vi "Create Execution Unit.vi"(8 "error in":errorcluster, 10 "Custom Device Ref":T2=18446744073709551615 format="%.0x", 11 "Execution Unit Factory Implementation in":refnum<class "Execution Unit Factory.lvclass">) -> (0 "error out":errorcluster, 1 "Asynchronous Execution Units":T1[](array[typedef]) {"ReadWrite Channels" format="%.0x"; "Outgoing Channels" format="%.0x"; "Incoming Channels" format="%.0x"}, 2 "Inline Execution Units":T1[](array[typedef]) {"ReadWrite Channels" format="%.0x"; "Outgoing Channels" format="%.0x"; "Incoming Channels" format="%.0x"}, 3 "Execution Unit Factory Implementation out":refnum<class "Execution Unit Factory.lvclass">)   [LabVIEW 2020, in "AIM ARINC 664 Engine.lvlib" / "Implementation.lvlib" / "Execution Unit Factory.lvclass"]
uses:
  Execution Unit Factory.lvclass
  <vilib>/NI VeriStand/Custom Device API/Custom Device Item Ref.ctl
  Interfaces/Controls/Execution Unit Information.ctl
  Interfaces/Execution Unit/Execution Unit.lvclass
  Tx Execution Unit/Tx Generic Execution Unit.lvclass
  C:/Users/Administrator/Desktop/GIT/niveristand-aim-arinc664-custom-device/Source/Custom Device Support/Engine/Interfaces/Execution Unit/Execution Unit.lvclass
  Tx UDP Execution Unit/Tx UDP Execution Unit.lvclass
  Rx UDP Execution Unit/Rx UDP Execution Unit.lvclass
  Monitor Execution Unit/Monitor Execution Unit.lvclass
  <vilib>/NI VeriStand/Custom Device API/Custom Device API.lvlib
  Interfaces/Interfaces.lvlib
  Scripting/AIM ARINC 664 Scripting.lvlib
  <vilib>/Utility/SystemLogging/NI_SystemLogging.lvlib
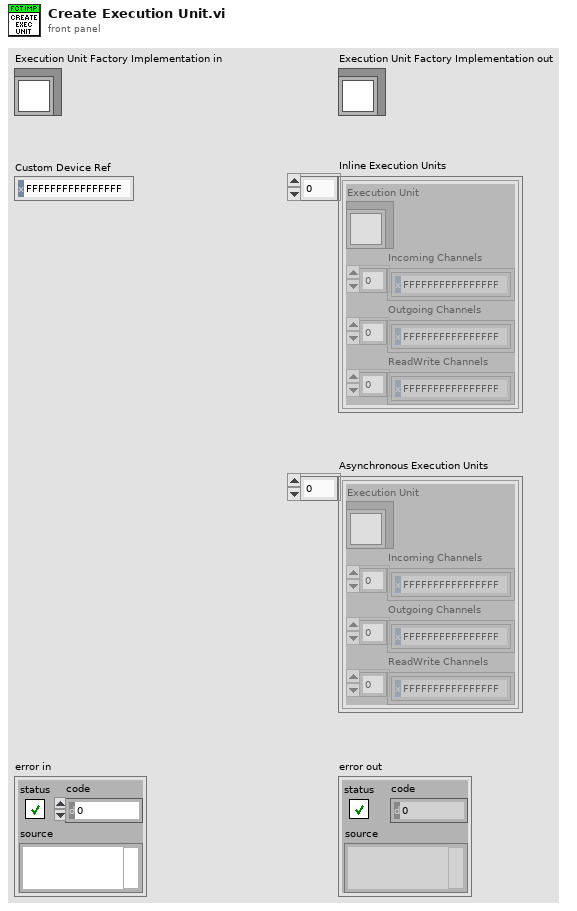
[diagram p1: front panel]
types:
  T1 = typedef "AIM ARINC 664 Engine.lvlib/Interfaces.lvlib/Execution Unit Information.ctl" = cluster{"Execution Unit":refnum<class "Execution Unit.lvclass">, "Incoming Channels":T2[], "Outgoing Channels":T2[], "ReadWrite Channels":T2[]}
  T2 = typedef "Custom Device API.lvlib/Custom Device Item Ref.ctl" = u64
  T3 = typedef "Custom Device API.lvlib/Custom Device Target Type.ctl" = enum16{"PharLap", "VxWorks", "Windows", "Linux_32_ARM", "Linux_x64"}
  T4 = typedef "AIM ARINC 664 Import.lvlib/board_setup.ctl" = cluster{"boardId":u32, "portSpeed":u32, "portConfig":u32}
  T5 = typedef "AIM ARINC 664 Import.lvlib/port_setup.ctl" = cluster{"port Id":u32, "redundant":bool}
  T6 = typedef "hardware_channels_tx.ctl" = cluster{"channel #":u16, "channel handle":u64, "InstrumentHandle_board":u32, "InstrumentHandle_port":u32, "channel settings":T7, "PayloadMap":map{string, u8[]}, "RawFrameMap":map{string, T10}}
  T7 = typedef "channel_settings_tx.ctl" = cluster{"Tx Board":u32, "Tx Port":u32, "Payload Parameter Array":T8[], "QueueSizeIn":u32, "Count":u32, "StartMode":u32}
  T8 = typedef "Frame Payload Parameters.ctl" = cluster{"PayloadID":string, "FrameIndeces":u32[], "Parameters":cluster{"start index":i32, "size":i32, "encoding":T9, "signed":bool, "scale multiplier":dbl, "scale offset":dbl}[]}
  T9 = typedef "Encoding (Arinc664).ctl" = u16
  T10 = typedef "RawFrame_entry.ctl" = cluster{"HeaderInfo":T11, "PayloadID":string}
  T11 = typedef "AIM664LV.lvlib/queue_header_generic.ctl" = cluster{"InterFrameGap":u32, "PacketGroupWaitTime":u32, "PayloadBufferMode":u8, "PayloadGenerationMode":u8, "PreambleCount":u8, "Skew":u32, "NetSelect":u8, "FrameStartMode":u8, "PhysErrorInjection":u32, "SequenceNumberInit":u16, "SequenceNumberOffset":u16}
  T12 = typedef "AIM664LV.lvlib/comm_config_vl_tx.ctl" = cluster{"VlId":u16, "NumOfSubVl":u16, "rate ms [Bag]":u32, "domainID":u8, "sideID":u8, "locationID":u8, "interfaceID":u8, "NetSelect":u32, "Skew":u32, "MaxFrameLength":u32, "FrameBufferSize":u32}
  T13 = typedef "AIM664LV.lvlib/comm_udp_tx.ctl" = cluster{"PortType":enum16{"FDX_UDP_SAMPLING", "FDX_UDP_QUEUING"}, "partitionID":u8, "SubVlId":u8, "UdpSrcPort":u16, "UdpDstPort":u16, "SampleRateMs":dbl, "UdpNumBufMessages":u32, "UdpMaxMessageSize":u32}
  T14 = cluster{"VL Config":T12, "CommPort Config":T13[]}[]
  T15 = cluster{"Data":u8[], "Parameters":cluster{"start index":i32, "size":i32, "encoding":T9, "signed":bool, "scale multiplier":dbl, "scale offset":dbl}[]}[]
  T16 = typedef "AIM664LV.lvlib/comm_verification_rx.ctl" = cluster{"VlId":u16, "VLRange":u32, "VerificationMode":u32, "Bag":u32, "Jitter":u32, "MaxFrameLength":u32, "MaxSkew":u32, "VLBufSize":u32, "FilterMode":u32, "FilterPosition":u32, "Padding":u32, "FilterMask":u32, "FilterData":u32, "MinFrameLength":u32}
  T17 = typedef "AIM664LV.lvlib/comm_udp_rx.ctl" = cluster{"PortType":enum16{"FDX_UDP_SAMPLING", "FDX_UDP_QUEUING"}, "SubVIId":u32, "domainID":u8, "sideID":u8, "locationID":u8, "partitionID":u8, "UdpSrcPort":u16, "UdpDstPort":u16, "UdpNumBufMessages":u32, "UdpMaxMessageSize":u32, "UdpSamplingRate":u32}
  T18 = cluster{"VL Config":T16, "CommPort Config":T17[]}[]
  T19 = typedef "rx_udp_payload_config.ctl" = cluster{"Data":u8[], "Parameters":cluster{"start index":i32, "size":i32, "encoding":T9, "signed":bool, "scale multiplier":dbl, "scale offset":dbl}[], "GetStatus":bool}
  T20 = typedef "loggingThreshold_types.ctl" = cluster{"Segmentation Threshold":dbl, "Disk Space Percentage":dbl, "Check Disk Space":bool, "Segment File":bool, "Segment Files By":u16}
  T21 = typedef "logFileInfo_types.ctl" = cluster{"Log Directory":string, "Base Name":string, "Timestamp":bool, "Enabled":bool}
  T22 = typedef "hardware_channels_rx.ctl" = cluster{"channel #":u16, "channel handle":u64, "InstrumentHandle_board":u32, "InstrumentHandle_port":u32, "Queue ID":u32, "channel settings":T23, "current log file name":path, "monitor queue settings":T25, "Log File Directory":string, "Base name":string, "Timestamp":bool, "log thresholds":T20}
  T23 = typedef "channel_settings_rx.ctl" = cluster{"Monitor Settings":T24, "Rx Board":u32, "Rx Port":u32}
  T24 = typedef "AIM664LV.lvlib/session_monitor_config.ctl" = cluster{"DefaultCronoMode":u32, "GlbMonBufferSizeIn":u32}
  T25 = typedef "monitor_queue_settings.ctl" = cluster{"TriggerPosition":u32, "CaptureMode":u32, "Strobe":u32, "MaxFileSize MB (1)":u32}
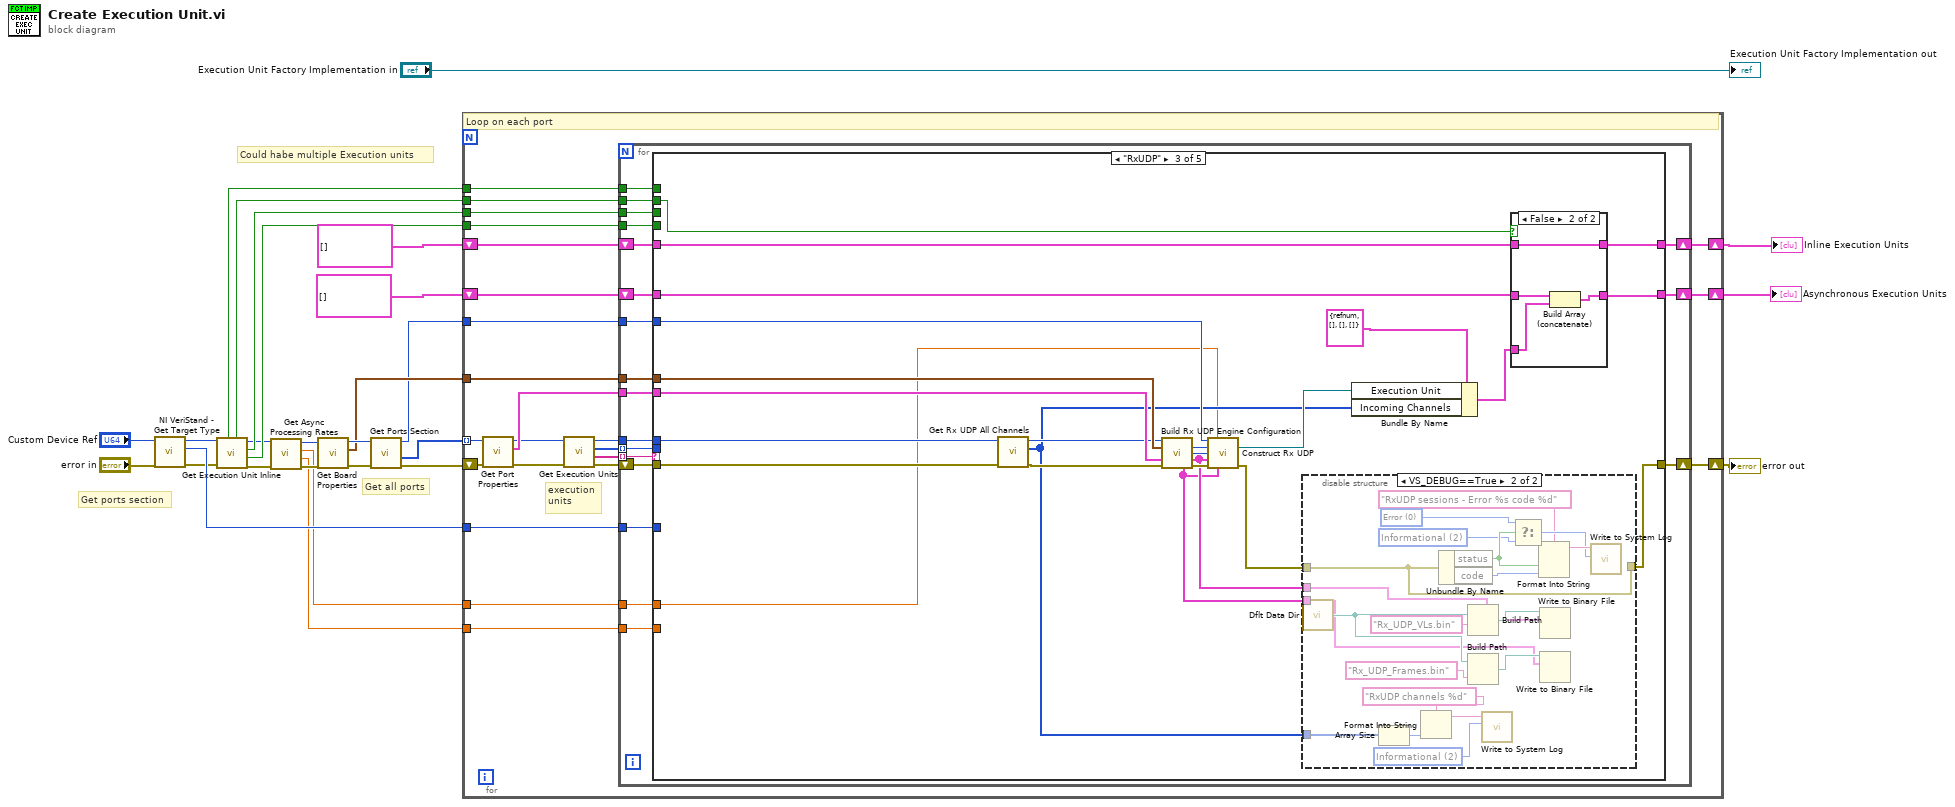
[diagram p0: block diagram]
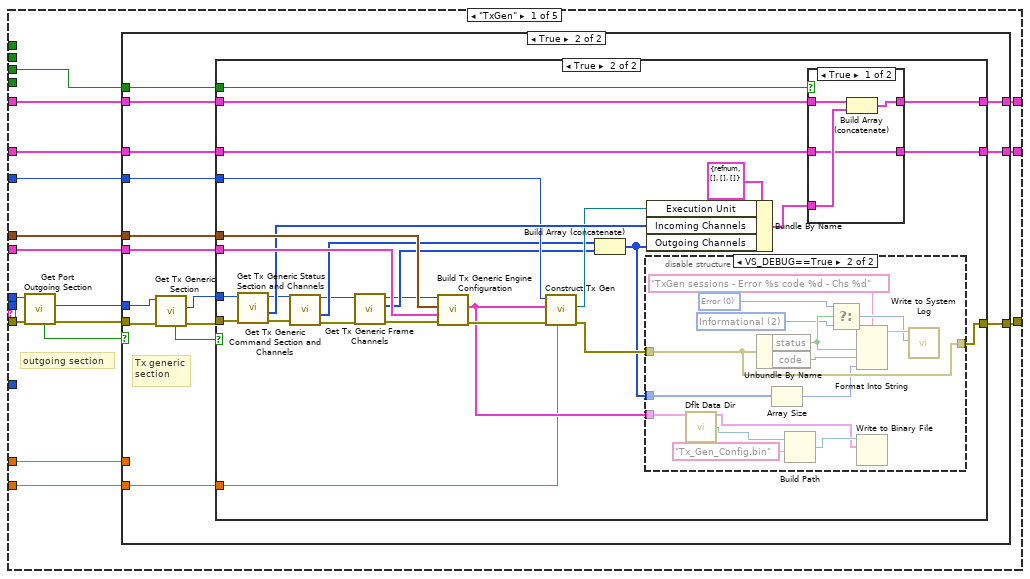
[diagram p2: hidden frame]
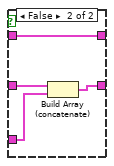
[diagram p5: hidden frame]
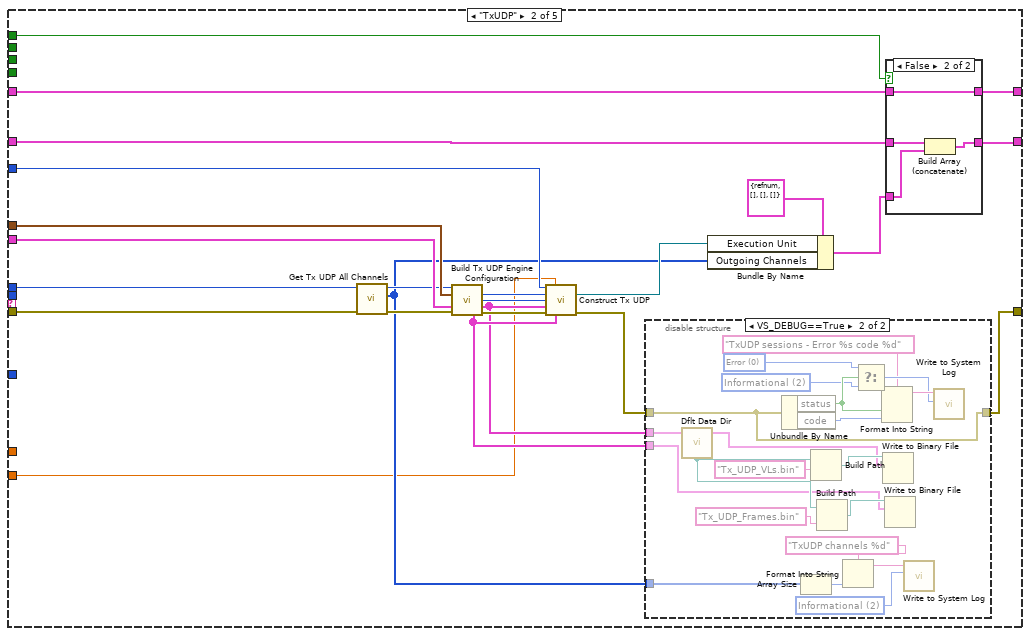
[diagram p7: hidden frame]
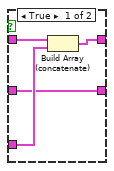
[diagram p8: hidden frame]
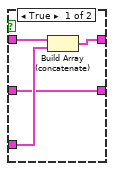
[diagram p10: hidden frame]
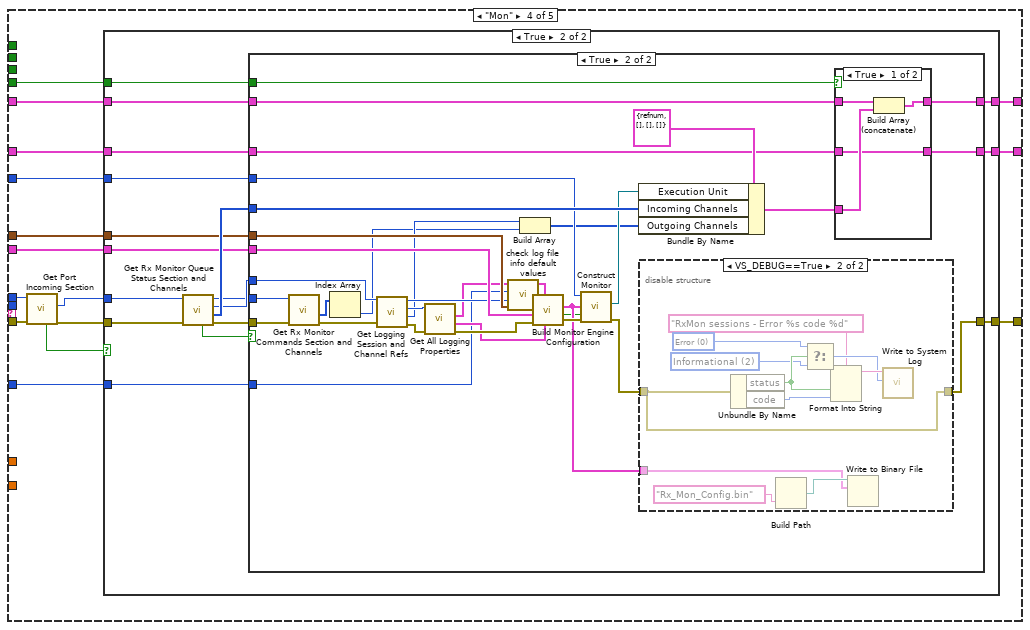
[diagram p12: hidden frame]
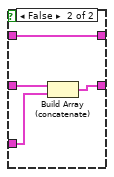
[diagram p15: hidden frame]
diagram:
  # "Get all ports"
  # "Get ports section"
  # "Could habe multiple Execution units"
  n1 = call <vilib>:"NI VeriStand - Get Target Type.vi"("error in (no error)"="error in", "Item Ref in"="Custom Device Ref") -> ("error out"=w12:errorcluster, "Target Type"=w13:T3, "Item Ref out"=w11:T2)  [unwired: 7 in]
  n2 = call "Get Execution Unit Inline.vi"("error in"=w12, "custom device ref"=w11) -> ("error out"=w5:errorcluster, "Inline Rx Execution"=w8:bool, "Inline Tx Generic"=w10:bool, "custom device ref out"=w6:T2, "Inline Rx UDP"=w7:bool, "Inline Tx UDP"=w9:bool)  [unwired: 4 in]
  n3 = call "Get Async Processing Rates.vi"("error in"=w5, "custom device ref"=w6) -> ("error out"=w4:errorcluster, "Outgoing Frame Rate"=w2:dbl, "Incoming Frame Rate"=w1:dbl, "custom device ref out"=w3:T2)  [unwired: 6 in]
  n4 = call "Get Board Properties.vi"("error in"=w4, "custom device ref"=w3) -> ("error out"=w21:errorcluster, "board properties out"=w19:T4, "custom device ref out"=w20:T2)  [unwired: 7 in]
  n5 = call "Get Ports Section.vi"("error in"=w21, "custom device ref"=w20) -> ("error out"=w18:errorcluster, "all ports refs out"=w17:T2[], "custom device ref out"=w16:T2)  [unwired: 6 in, 1 out]
  n6 = for {
    shift-right: [w46] -> w26
    shift-left: w18 -> [w43]
    tunnel: w17 -> [w44] mode=indexing
    shift-right: [w48] -> w22
    shift-left: T1[] [] ("Array") -> [w49]
    shift-right: [w47] -> w23
    shift-left: T1[] [] ("Array") -> [w50]
    tunnel: w19 -> [w45]
    tunnel: w16 -> [w41]
    tunnel: w13 -> [w34]
    tunnel: w10 -> [w33]
    tunnel: w9 -> [w32]
    tunnel: w8 -> [w31]
    tunnel: w7 -> [w30]
    tunnel: w2 -> [w29]
    tunnel: w1 -> [w28]
    # "execution\nunits"
    # "Loop on each port"
    n7 = call "Get Port Properties.vi"("error in"=w43, "custom device ref"=w44) -> ("error out"=w39:errorcluster, "port properties out"=w42:T5, "custom device ref out"=w40:T2)  [unwired: 7 in]
    n8 = call "Get Execution Units.vi"("error in"=w39, "custom device ref"=w40) -> ("error out"=w37:errorcluster, "List of Execution Units"=w35:string[], "Execution Units Refs"=w36:T2[], "custom device ref out"=w38:T2)  [unwired: 6 in]
    n9 = for {
      tunnel: w38 -> [w68]
      shift-right: [w63] -> w46
      shift-left: w37 -> [w69]
      shift-right: [w64] -> w47
      shift-left: w50 -> [w67]
      shift-right: [w65] -> w48
      shift-left: w49 -> [w66]
      tunnel: w42 -> [w62]
      tunnel: w45 -> [w61]
      tunnel: w41 -> [w60]
      tunnel: w36 -> [w58] mode=indexing
      tunnel: w35 -> [w59] mode=indexing
      tunnel: w34 -> [w57]
      tunnel: w33 -> [w56]
      tunnel: w32 -> [w55]
      tunnel: w31 -> [w54]
      tunnel: w30 -> [w53]
      tunnel: w29 -> [w52]
      tunnel: w28 -> [w51]
      n10 = case shown="\"RxUDP\"" w59 {
        tunnel: w69 -> [w85 w181 w234 w278 w355]
        tunnel: w68 -> [w84 w170 w223 w277 _]
        tunnel: w67 -> [w80 w162 w216 w273 w357]
        tunnel: w66 -> [w79 w164 w214 w272 w356]
        tunnel: [w77 w159 w213 w271 w356] -> w65
        tunnel: [w78 w160 w217 w270 w357] -> w64
        tunnel: [w76 w166 w219 w269 w355] -> w63
        tunnel: w62 -> [w75 w175 w228 w267 _]
        tunnel: w61 -> [w74 w176 w229 w268 _]
        tunnel: w60 -> [w73 w171 w224 w266 _]
        tunnel: w58 -> [_ _ _ _ _]
        tunnel: w57 -> [_ _ _ w265 _]
        tunnel: w56 -> [w72 _ _ _ _]
        tunnel: w55 -> [_ w161 _ _ _]
        tunnel: w54 -> [_ _ _ w264 _]
        tunnel: w53 -> [_ _ w212 _ _]
        tunnel: w52 -> [w71 w158 _ _ _]
        tunnel: w51 -> [w70 _ w211 _ _]
        frame "TxGen" {
          # "outgoing section"
          n11 = call "Get Port Outgoing Section.vi"("error in"=w85, "ports ref"=w84) -> ("error out"=w82:errorcluster, "outgoing section ref out"=w81:T2, "found?"=w83:bool)  [unwired: 6 in, 1 out]
          n12 = case shown="True" w83 {
            tunnel: w82 -> [w86 w96]
            tunnel: w81 -> [_ w95]
            tunnel: w80 -> [w88 w102]
            tunnel: w79 -> [w87 w101]
            tunnel: [w88 w103] -> w78
            tunnel: [w87 w100] -> w77
            tunnel: [w86 w99] -> w76
            tunnel: w75 -> [_ w98]
            tunnel: w74 -> [_ w97]
            tunnel: w73 -> [_ w91]
            tunnel: w72 -> [_ w90]
            tunnel: w71 -> [_ w89]
            tunnel: w70 -> [_ _]
            frame False {
            }
            frame True {
              # "Tx generic\nsection"
              n13 = call "Get Tx Generic Section.vi"("error in"=w96, "Parent section Ref in"=w95) -> ("error out"=w93:errorcluster, "Item Ref"=w92:T2, "found?"=w94:bool)  [unwired: 6 in, 1 out]
              n14 = case shown="True" w94 {
                tunnel: w93 -> [w104 w128]
                tunnel: [w106 w112] -> w103
                tunnel: w102 -> [w106 w133]
                tunnel: w101 -> [w105 w132]
                tunnel: [w105 w110] -> w100
                tunnel: [w104 w118] -> w99
                tunnel: w98 -> [_ w130]
                tunnel: w97 -> [_ w129]
                tunnel: w92 -> [_ w127]
                tunnel: w91 -> [_ w124]
                tunnel: w90 -> [_ w108]
                tunnel: w89 -> [_ w107]
                frame False {
                }
                frame True {
                  n15 = call "Get Tx Generic Status Section and Channels.vi"("error in"=w128, "Tx generic ref"=w127) -> ("error out"=w122:errorcluster, "Tx generic status channel refs"=w126:T2[], "Tx generic ref out"=w123:T2)  [unwired: 5 in, 2 out]
                  n16 = call "Get Tx Generic Command Section and Channels.vi"("error in"=w122, "Tx generic ref"=w123) -> ("error out"=w117:errorcluster, "Tx generic command channel refs"=w121:T2[], "Tx generic ref out"=w116:T2)  [unwired: 5 in, 2 out]
                  n17 = call "Get Tx Generic Frame Channels.vi"("error in"=w117, "Tx generic ref"=w116) -> ("error out"=w115:errorcluster, "Tx generic frame channels"=w114:T2[], "Tx generic ref out"=w113:T2)  [unwired: 6 in, 1 out]
                  n18 = call "Build Tx Generic Engine Configuration.vi"("error in"=w115, "port properties"=w130, "board properties"=w129, "section ref in"=w113) -> ("error out"=w131:errorcluster, "Tx cluster out"=w119:T6)  [unwired: 5 in, 1 out]
                  n19 = call "Construct Tx Gen.vi"("async loop rate hz"=w107, "error in (no error)"=w131, "TX Parameters"=w119, "custom device ref in"=w124) -> ("error out"=w120:errorcluster, "Tx Execution Unit out"=w125:refnum<class "Tx Generic Execution Unit.lvclass">)  [unwired: 4 in, 1 out]
                  n20 = Build Array (concatenate)(w121, w114) -> (w111:T2[])
                  n21 = disable-structure shown="VS_DEBUG==True" {
                    disable-tunnel: w120 -> [w143 w146]
                    disable-tunnel: w119 -> [_ w147]
                    disable-tunnel: [w143 w146] -> w118
                    disable-tunnel: w111 -> [_ w145]
                    frame condition #0 (active) {
                    }
                    frame condition #1 {
                      w153 = 2 items=["Error", "Warning", "Informational"] ("severity")
                      w154 = 0 items=["Error", "Warning", "Informational"] ("severity")
                      n22 = call <vilib>:"Dflt Data Dir.vi"() -> ("App:Default Data Directory"=w150:path)
                      n23 = Unbundle By Name(w146) -> ("status"=w155:bool, "code"=w156:i32)
                      n24 = Array Size(array=w145) -> (size(s)=w144:i32)
                      n25 = Build Path(base path=w150, name or relative path="Tx_Gen_Config.bin" ("format string")) -> (appended path=w148:path)
                      n26 = Select(t=w154, s=w155, f=w153) -> (s? t:f=w152:i32)
                      n27 = Format Into String(format string="TxGen sessions - Error %s code %d - Chs %d", w155, w156, w144) -> (resulting string=w157:string)  [unwired: 2 in, 1 out]
                      n28 = Write to Binary File(file (use dialog)=w148, data=w147) -> ()  [unwired: 4 in, 3 out]
                      n29 = call <vilib>:"Write to System Log.vi"("severity"=w152, "message"=w157) -> ()  [unwired: 9 in, 1 out]
                    }
                  }
                  n30 = Bundle By Name(cluster=T1 {"Execution Unit"=refnum, "Incoming Channels"=[], "Outgoing Channels"=[], "ReadWrite Channels"=[]} ("Execution Unit Information"), "Execution Unit"=w125, "Incoming Channels"=w126, "Outgoing Channels"=w111) -> (w109:T1)
                  n31 = case shown="True" w108 {
                    tunnel: w133 -> [w138 w142]
                    tunnel: w132 -> [w135 w141]
                    tunnel: [w137 w142] -> w112
                    tunnel: [w135 w140] -> w110
                    tunnel: w109 -> [w136 w139]
                    frame True {
                      n32 = Build Array (concatenate)(w138, w136) -> (w137:T1[])
                    }
                    frame False {
                      n33 = Build Array (concatenate)(w141, w139) -> (w140:T1[])
                    }
                  }
                }
              }
            }
          }
        }
        frame "TxUDP" {
          n34 = call "Get Tx UDP All Channels.vi"("error in"=w181, "custom device ref in"=w170) -> ("error out"=w178:errorcluster, "Tx UDP channel refs out"=w165:T2[], "custom device ref out"=w172:T2)  [unwired: 7 in]
          n35 = call "Build Tx UDP Engine Configuration.vi"("section ref in"=w172, "board properties"=w176, "port properties"=w175, "error in"=w178) -> ("boardId"=w174:u32, "portId"=w173:u32, "VL configurations"=w167:T14, "comm port payload"=w168:T15, "error out"=w177:errorcluster)  [unwired: 6 in, 1 out]
          n36 = call "Construct Tx UDP.vi"("custom device ref in"=w171, "async loop rate hz"=w158, "InstrumentHandle_board"=w174, "InstrumentHandle_port"=w173, "VL Configurations"=w167, "error in (no error)"=w177, "CommPort Payload"=w168) -> ("Execution Unit Out"=w179:refnum<class "Tx UDP Execution Unit.lvclass">, "error out"=w169:errorcluster)  [unwired: 6 in, 1 out]
          n37 = disable-structure shown="VS_DEBUG==True" {
            disable-tunnel: w169 -> [w190 w196]
            disable-tunnel: w168 -> [_ w197]
            disable-tunnel: w167 -> [_ w198]
            disable-tunnel: [w190 w196] -> w166
            disable-tunnel: w165 -> [_ w193]
            frame condition #0 (active) {
            }
            frame condition #1 {
              w191 = 2 items=["Error", "Warning", "Informational"] ("severity")
              w206 = 2 items=["Error", "Warning", "Informational"] ("severity")
              w207 = 0 items=["Error", "Warning", "Informational"] ("severity")
              n38 = call <vilib>:"Dflt Data Dir.vi"() -> ("App:Default Data Directory"=w203:path)
              n39 = Unbundle By Name(w196) -> ("status"=w208:bool, "code"=w209:i32)
              n40 = Array Size(array=w193) -> (size(s)=w195:i32)
              n41 = Build Path(base path=w203, name or relative path="Tx_UDP_VLs.bin" ("format string")) -> (appended path=w200:path)
              n42 = Build Path(base path=w203, name or relative path="Tx_UDP_Frames.bin" ("format string")) -> (appended path=w199:path)
              n43 = Format Into String(format string="TxUDP channels %d", w195) -> (resulting string=w194:string)  [unwired: 2 in, 1 out]
              n44 = Select(t=w207, s=w208, f=w206) -> (s? t:f=w205:i32)
              n45 = Format Into String(format string="TxUDP sessions - Error %s code %d", w208, w209) -> (resulting string=w210:string)  [unwired: 2 in, 1 out]
              n46 = Write to Binary File(file (use dialog)=w200, data=w198) -> ()  [unwired: 4 in, 3 out]
              n47 = Write to Binary File(file (use dialog)=w199, data=w197) -> ()  [unwired: 4 in, 3 out]
              n48 = call <vilib>:"Write to System Log.vi"("severity"=w191, "message"=w194) -> ()  [unwired: 9 in, 1 out]
              n49 = call <vilib>:"Write to System Log.vi"("severity"=w205, "message"=w210) -> ()  [unwired: 9 in, 1 out]
            }
          }
          n50 = Bundle By Name(cluster=T1 {"Execution Unit"=refnum, "Incoming Channels"=[], "Outgoing Channels"=[], "ReadWrite Channels"=[]} ("Execution Unit Information"), "Execution Unit"=w179, "Outgoing Channels"=w165) -> (w163:T1)
          n51 = case shown="False" w161 {
            tunnel: w162 -> [w185 w189]
            tunnel: w164 -> [w182 w188]
            tunnel: [w184 w189] -> w160
            tunnel: [w182 w187] -> w159
            tunnel: w163 -> [w183 w186]
            frame True {
              n52 = Build Array (concatenate)(w185, w183) -> (w184:T1[])
            }
            frame False {
              n53 = Build Array (concatenate)(w188, w186) -> (w187:T1[])
            }
          }
        }
        frame "RxUDP" {
          n54 = call "Get Rx UDP All Channels.vi"("error in"=w234, "custom device ref in"=w223) -> ("error out"=w231:errorcluster, "Rx UDP channel refs"=w218:T2[], "custom device ref out"=w225:T2)  [unwired: 7 in]
          n55 = call "Build Rx UDP Engine Configuration.vi"("section ref in"=w225, "board properties"=w229, "port properties"=w228, "error in"=w231) -> ("boardId"=w227:u32, "portId"=w226:u32, "VL Configurations"=w222:T18, "CommPort Payload"=w221:T19[], "error out"=w230:errorcluster)  [unwired: 6 in, 1 out]
          n56 = call "Construct Rx UDP.vi"("custom device ref in"=w224, "async loop rate hz"=w211, "InstrumentHandle_board"=w227, "InstrumentHandle_port"=w226, "VL Configurations"=w222, "error in (no error)"=w230, "CommPort Payload"=w221) -> ("Execution Unit Out"=w232:refnum<class "Rx UDP Execution Unit.lvclass">, "error out"=w220:errorcluster)  [unwired: 6 in, 1 out]
          n57 = disable-structure shown="VS_DEBUG==True" {
            disable-tunnel: w220 -> [w243 w249]
            disable-tunnel: w221 -> [_ w250]
            disable-tunnel: w222 -> [_ w251]
            disable-tunnel: [w243 w249] -> w219
            disable-tunnel: w218 -> [_ w244]
            frame condition #0 (active) {
            }
            frame condition #1 {
              w245 = 2 items=["Error", "Warning", "Informational"] ("severity")
              w259 = 2 items=["Error", "Warning", "Informational"] ("severity")
              w260 = 0 items=["Error", "Warning", "Informational"] ("severity")
              n58 = call <vilib>:"Dflt Data Dir.vi"() -> ("App:Default Data Directory"=w256:path)
              n59 = Array Size(array=w244) -> (size(s)=w248:i32)
              n60 = Format Into String(format string="RxUDP channels %d", w248) -> (resulting string=w247:string)  [unwired: 2 in, 1 out]
              n61 = Unbundle By Name(w249) -> ("status"=w261:bool, "code"=w262:i32)
              n62 = Build Path(base path=w256, name or relative path="Rx_UDP_VLs.bin" ("format string")) -> (appended path=w253:path)
              n63 = Build Path(base path=w256, name or relative path="Rx_UDP_Frames.bin" ("format string")) -> (appended path=w252:path)
              n64 = call <vilib>:"Write to System Log.vi"("severity"=w245, "message"=w247) -> ()  [unwired: 9 in, 1 out]
              n65 = Select(t=w260, s=w261, f=w259) -> (s? t:f=w258:i32)
              n66 = Format Into String(format string="RxUDP sessions - Error %s code %d", w261, w262) -> (resulting string=w263:string)  [unwired: 2 in, 1 out]
              n67 = Write to Binary File(file (use dialog)=w253, data=w251) -> ()  [unwired: 4 in, 3 out]
              n68 = Write to Binary File(file (use dialog)=w252, data=w250) -> ()  [unwired: 4 in, 3 out]
              n69 = call <vilib>:"Write to System Log.vi"("severity"=w258, "message"=w263) -> ()  [unwired: 9 in, 1 out]
            }
          }
          n70 = Bundle By Name(cluster=T1 {"Execution Unit"=refnum, "Incoming Channels"=[], "Outgoing Channels"=[], "ReadWrite Channels"=[]} ("Execution Unit Information"), "Execution Unit"=w232, "Incoming Channels"=w218) -> (w215:T1)
          n71 = case shown="False" w212 {
            tunnel: w216 -> [w238 w242]
            tunnel: w214 -> [w235 w239]
            tunnel: [w237 w242] -> w217
            tunnel: [w235 w241] -> w213
            tunnel: w215 -> [w236 w240]
            frame True {
              n72 = Build Array (concatenate)(w238, w236) -> (w237:T1[])
            }
            frame False {
              n73 = Build Array (concatenate)(w239, w240) -> (w241:T1[])
            }
          }
        }
        frame "Mon" {
          n74 = call "Get Port Incoming Section.vi"("error in"=w278, "ports ref"=w277) -> ("error out"=w275:errorcluster, "incoming ref out"=w274:T2, "found?"=w276:bool)  [unwired: 6 in, 1 out]
          n75 = case shown="True" w276 {
            tunnel: w275 -> [w281 w285]
            tunnel: w274 -> [_ w287]
            tunnel: w273 -> [w279 w296]
            tunnel: w272 -> [w280 w295]
            tunnel: [w280 w293] -> w271
            tunnel: [w279 w292] -> w270
            tunnel: [w281 w291] -> w269
            tunnel: w268 -> [_ w290]
            tunnel: w267 -> [_ w289]
            tunnel: w266 -> [_ w286]
            tunnel: w265 -> [_ w283]
            tunnel: w264 -> [_ w282]
            frame False {
            }
            frame True {
              n76 = call "Get Rx Monitor Queue Status Section and Channels.vi"("error in"=w285, "custom device ref in"=w287) -> ("error out"=w297:errorcluster, "Rx monitor section channel refs"=w294:T2[], "Rx monitor section ref out"=w288:T2, "custom device ref out"=w284:T2, "found?"=w298:bool)  [unwired: 5 in]
              n77 = case shown="True" w298 {
                tunnel: w297 -> [w299 w317]
                tunnel: w296 -> [w301 w307]
                tunnel: w295 -> [w300 w305]
                tunnel: w294 -> [_ w330]
                tunnel: [w300 w304] -> w293
                tunnel: [w301 w306] -> w292
                tunnel: [w299 w319] -> w291
                tunnel: w288 -> [_ w315]
                tunnel: w290 -> [_ w332]
                tunnel: w289 -> [_ w331]
                tunnel: w286 -> [_ w328]
                tunnel: w284 -> [_ w314]
                tunnel: w283 -> [_ w308]
                tunnel: w282 -> [_ w302]
                frame False {
                }
                frame True {
                  n78 = call "Get Rx Monitor Commands Section and Channels.vi"("error in"=w317, "custom device ref in"=w314) -> ("error out"=w316:errorcluster, "Rx monitor section channel refs"=w312:T2[])  [unwired: 5 in, 3 out]
                  n79 = Index Array(array=w312) -> (element=w311:T2)  [unwired: 1 in]
                  n80 = call "Get Logging Session and Channel Refs.vi"("error in"=w316, "secton ref in"=w315) -> ("error out"=w325:errorcluster, "Channel Ref"=w313:T2, "logging"=w326:T2, "section ref out"=w327:T2)  [unwired: 6 in]
                  n81 = call "Get All Logging Properties.vi"("error in"=w325, "logging ref"=w326) -> ("error out"=w324:errorcluster, "log thresholds"=w323:T20, "log file info"=w322:T21)  [unwired: 6 in, 1 out]
                  n82 = call "check log file info default values.vi"("Target Type"=w308, "log file info in"=w322) -> ("log file info out"=w321:T21)  [unwired: 9 in]
                  n83 = Build Array(w313, w311) -> (w310:T2[])
                  n84 = call "Build Monitor Engine Configuration.vi"("log thresholds"=w323, "log file info"=w321, "error in"=w324, "port properties"=w331, "board properties"=w332, "section ref in"=w327) -> ("error out"=w334:errorcluster, "Enabled"=w309:bool, "Monitor cluster out"=w318:T22)  [unwired: 2 in, 1 out]
                  n85 = call "Construct Monitor.vi"("error in (no error)"=w334, "Enable Logging?"=w309, "Monitor Parameters"=w318, "custom device ref in"=w328) -> ("error out"=w320:errorcluster, "Monitor Execution Unit out"=w329:refnum<class "Monitor Execution Unit.lvclass">)  [unwired: 4 in, 1 out]
                  n86 = Bundle By Name(cluster=T1 {"Execution Unit"=refnum, "Incoming Channels"=[], "Outgoing Channels"=[], "ReadWrite Channels"=[]} ("Execution Unit Information"), "Execution Unit"=w329, "Incoming Channels"=w330, "Outgoing Channels"=w310) -> (w303:T1)
                  n87 = disable-structure shown="VS_DEBUG==True" {
                    disable-tunnel: w320 -> [w343 w345]
                    disable-tunnel: [w343 w345] -> w319
                    disable-tunnel: w318 -> [_ w344]
                    frame condition #0 (active) {
                    }
                    frame condition #1 {
                      w350 = 2 items=["Error", "Warning", "Informational"] ("severity")
                      w351 = 0 items=["Error", "Warning", "Informational"] ("severity")
                      n88 = Unbundle By Name(w345) -> ("status"=w352:bool, "code"=w353:i32)
                      n89 = Build Path(name or relative path="Rx_Mon_Config.bin" ("format string")) -> (appended path=w346:path)  [unwired: 1 in]
                      n90 = Select(t=w351, s=w352, f=w350) -> (s? t:f=w349:i32)
                      n91 = Format Into String(format string="RxMon sessions - Error %s code %d", w352, w353) -> (resulting string=w354:string)  [unwired: 2 in, 1 out]
                      n92 = Write to Binary File(file (use dialog)=w346, data=w344) -> ()  [unwired: 4 in, 3 out]
                      n93 = call <vilib>:"Write to System Log.vi"("severity"=w349, "message"=w354) -> ()  [unwired: 9 in, 1 out]
                    }
                  }
                  n94 = case shown="True" w302 {
                    tunnel: w307 -> [w338 w342]
                    tunnel: w305 -> [w335 w341]
                    tunnel: [w337 w342] -> w306
                    tunnel: [w335 w340] -> w304
                    tunnel: w303 -> [w336 w339]
                    frame True {
                      n95 = Build Array (concatenate)(w338, w336) -> (w337:T1[])
                    }
                    frame False {
                      n96 = Build Array (concatenate)(w341, w339) -> (w340:T1[])
                    }
                  }
                }
              }
            }
          }
        }
        frame Default {
        }
      }
    }
  }
  "error out" <- w26
  "Inline Execution Units" <- w23
  "Asynchronous Execution Units" <- w22
  "Execution Unit Factory Implementation out" <- "Execution Unit Factory Implementation in"
